vi "Nicolet 12 ICAI_gatefix4.vi"(3 "?":u16(ring)=10 items=["16", "32", "64", "128", "256", "512", "1024", "2048", "4096", "8192", "16384", "32768", "65536", "131072", "262144", "524288 (one channel)", ""], 5 "Sample Duration (sec)":u32(knob)=24 scale=1.0..33.0) -> (0 "Waveform Graph":waveform(dbl)[](graph)=[{"t0"=timestamp(0 s since 1904-01-01), "dt"=0.0001220703125, "Y"=array[40960 elements]}, {"t0"=timestamp(0 s since 1904-01-01), "dt"=0.0001220703125, "Y"=array[40960 elements]}], 2 "data":dbl[][](array[numeric]) format="%0.2f", 8 "points":i32=40960)   [LabVIEW 2010]
doc: "I. Description:\nThis example demonstrates how to acquire a finite amount of data (Waveform) using the DAQ device's internal clock, started by an analog edge condition.\n\nII. Instructions for Running:\n1. Select the physical channel to correspond to where your signal is input on the DAQ device.\n2. Enter the minimum and maximum voltage range.\nNote: For better accuracy try to match the input range to the expected voltage level of the measured signal.\n3. Set the number of samples to acquire per channel.\n4. Set the rate of the acquisition\nNote: The rate should be AT LEAST twice as fast as the maximum frequency component of the signal being acquired.\n5. Set the source of the start trigger. By default this is PFI0\n6. Set the slope and level of desired analog edge condition.\n\nIII. Block Diagram Steps:\n1. Create an empty task.\n2. Create an analog input voltage channel.\n3. Set the rate for the sample clock. Additionally, define the sample mode to be finite.\n4. Define the parameters for an Analog Slope Start Trigger.\n5. Call the Start VI to start the acquisition.\n6. Read all of the data.\n7. Stop the Analog Input Task.\n8. Call the Clear Task VI to clear the Task.\n9. Use the popup dialog box to display an error if any\nIV. I/O Connections Overview:\nMake sure your signal input terminal matches the Physical Channel I/O Control. In this case wire your signal to the ai0 pin on your DAQ Device."
uses:
  programs/Detection/200262.llb/Trigger Select.ctl
  <vilib>/Utility/error.llb/DialogType.ctl
  <vilib>/DAQmx/read.llb/DAQmx Read (Analog 2D DBL NChan NSamp).vi
  <vilib>/DAQmx/create/channels.llb/DAQmx Create Channel (AI-Voltage-Basic).vi
  <vilib>/DAQmx/configure/timing.llb/DAQmx Timing (Sample Clock).vi
  <vilib>/DAQmx/configure/trigger.llb/DAQmx Start Trigger (Analog Edge).vi
  <vilib>/DAQmx/configure/trigger.llb/DAQmx Reference Trigger (Digital Edge).vi
  <vilib>/daqmx/miscellaneous.llb/DAQmx Fill In Error Info.vi
  Program Files/National Instruments/LabVIEW 2010/resource/objmgr/daqmx.rc
  <instrlib>/BK Precision 911X Series/BK Precision 911X Series.lvlib
panel:
  in  "Final Current":dbl=16.5
  in  "Current Step (0.0A":dbl=0.02
  in  "Starting Current (0.0 A)":dbl=18.0 format="%.3g"
  in  "Voltage Level (0.0 V)":dbl=15.0 format="%.3f"
  in  "Enable OVP (T: Enable)":bool=TRUE
  in  "Voltage Limit (0V)":dbl=25.0 format="%.2f"
  in  "Magnet Supply VISA name":refnum<visa-resource-name>="GPIB0::1::INSTR"
  out "size(s)":i32[](array[numeric])
  in  "CAI/ICAI":bool=TRUE
  in  "?":path=path "C:/Users/Cardenas/Desktop/7_01/7_01_380fringe371mvmid_lockedat330.txt"
  in  "Path":path=path "C:/Users/Cardenas/Desktop/Feb_2026/02_13_17Mhz_18a_start_p005fall_500uVsense_10avgs_1750hzcenter_negslope.txt"
  out "Time":dbl=5.5
  out "points pretriger":dbl=4096.0
  in  "Iterations to Average":i32=10
  in  "Sample Rate Hz":bool
  out "Cursor Time Selected":dbl=0.22413589186805782
  out "Cursor Peak to Peak Voltage":dbl=0.01024955436720143
  in  "Save Average To File":bool
  out "Pretrigger Samples":dbl=4096.0
  out "Seconds Per Division":dbl=0.1
  out "Posttrigger Samples Captured":dbl=40960.0
  in  "Voltage Offset":dbl(knob) scale=-2.0..2.0
  in  "Average / Live Display":bool
  in  "Seconds  Per Division":u32(knob) min=1 max=1 step=1 scale=0.0..15.0
  out "Samples Averaged":i32=3
  in  "?":bool=TRUE
  in  "Volts Per Division":dbl(knob)=0.5 scale=0.005..5.0
  in  "Pretrigger Duration (%)":dbl(knob)=0.1 min=0.0 max=2.0 step=1.0 scale=0.05..0.95
  in  "Analog Source":string="APFI0"
  in  "Digital External TTL Source":tag="/Dev1/PFI13"
  in  "Trigger Type":T1=enum."Digital Edge"
  in  "Analog Edge Level":dbl=-0.1 format="%0.2f"
  in  "Edge":i32(ring)=10280 items=["Rising"=10280, "Falling"=10171]
  in  "Physical Channel":tag="Dev1/ai22, Dev1/ai23" caption="Physical Channels"
  out "Sampling Iterations":i32=2
  in  "Maximum  Voltage":dbl=10.0
  in  "Minimum Voltage":dbl=-10.0
  out "Sampling Rate":i32=8192 caption="Sample Rate (Hz)"
  in  "stop":bool
  # "Channel\nConfiguration"
  # "Triggering Parameters"
  # "Voltage Parameters"
  # "TTL Trigger Options"
  # "Timing Parameters"
  # "External  Trigger Options"
  # "Storage Options"
  # "Nicolet 8.vi*If X scale markers are not drawn:\nRight click the waveform diagram -> select X axis -> marker spacing -> set to arbitrary AFTER\nsetting the correct seconds per division"
  # "CAI / ICAI"
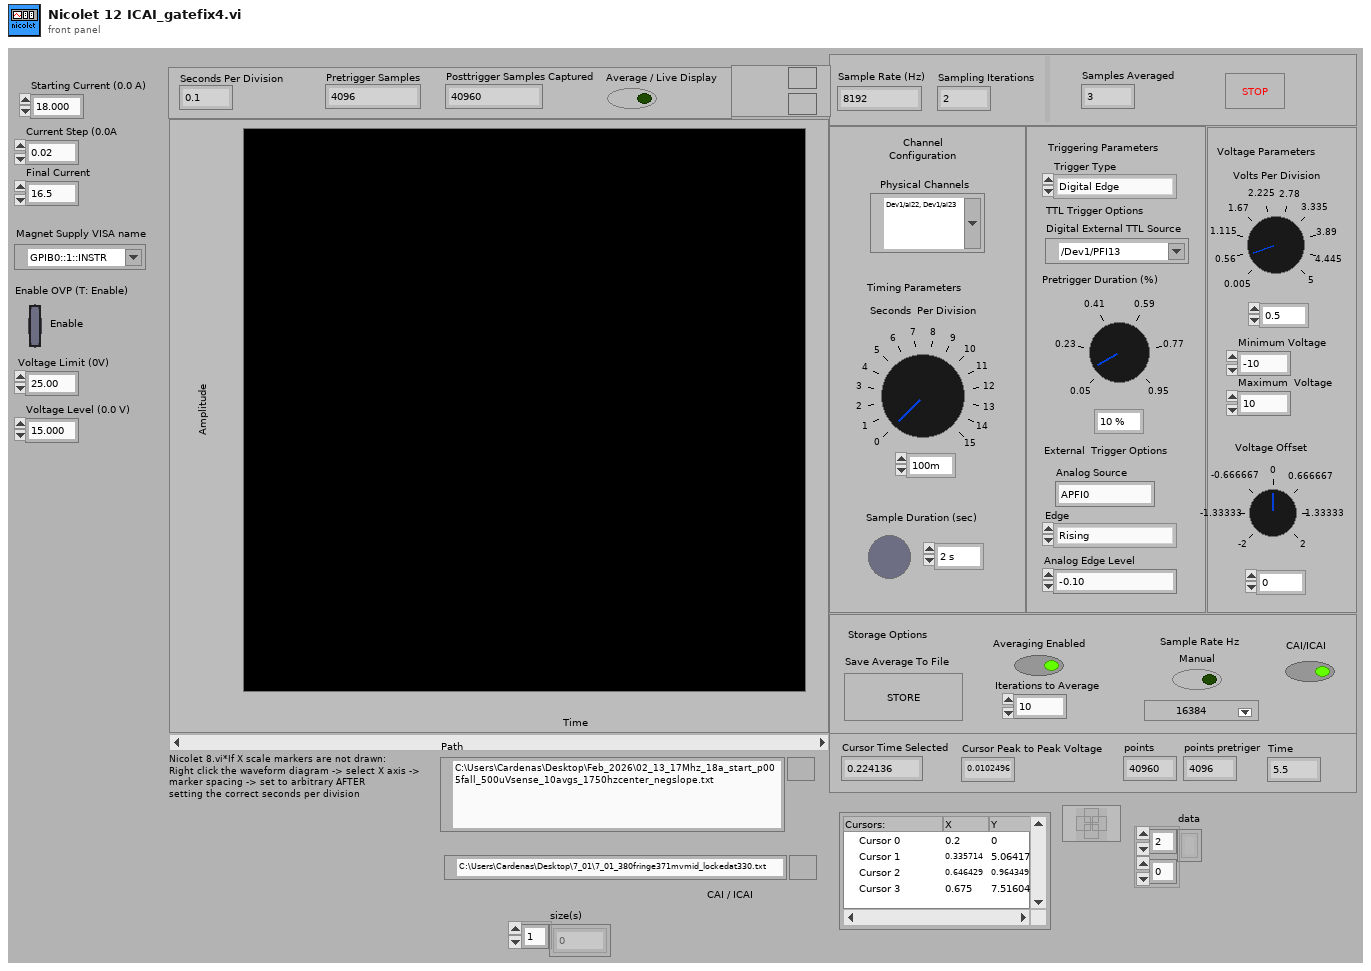
[diagram p1: front panel]
types:
  T1 = typedef "Trigger Select.ctl" = enum16{"None", "Analog Edge", "Digital Edge"}
  T2 = typedef "DialogType.ctl" = u16
  T3 = typedef "LVCursorListTypeDef.ctl" = cluster{"Name":string, "Color":u32, "Style":u8, "Point Style":u8, "Name Visible":bool, "Allow Drag":bool, "Cursor Mode":u32, "Plot":i32, "Index":i32, "Position":cluster{"X":dbl, "Y":dbl}, "X Scale":u32, "Y Scale":u32, "Watch Plots":i32[], "Watch All Plots":bool, "Plot Area":i32, "Label Offset":cluster{"X":dbl, "Y":dbl}}[]
  T4 = cluster{"Name":string, "Color":u32, "Style":u8, "Point Style":u8, "Name Visible":bool, "Allow Drag":bool, "Cursor Mode":u32, "Plot":i32, "Index":i32, "Position":cluster{"X":dbl, "Y":dbl}, "X Scale":u32, "Y Scale":u32, "Watch Plots":i32[], "Watch All Plots":bool, "Plot Area":i32, "Label Offset":cluster{"X":dbl, "Y":dbl}}
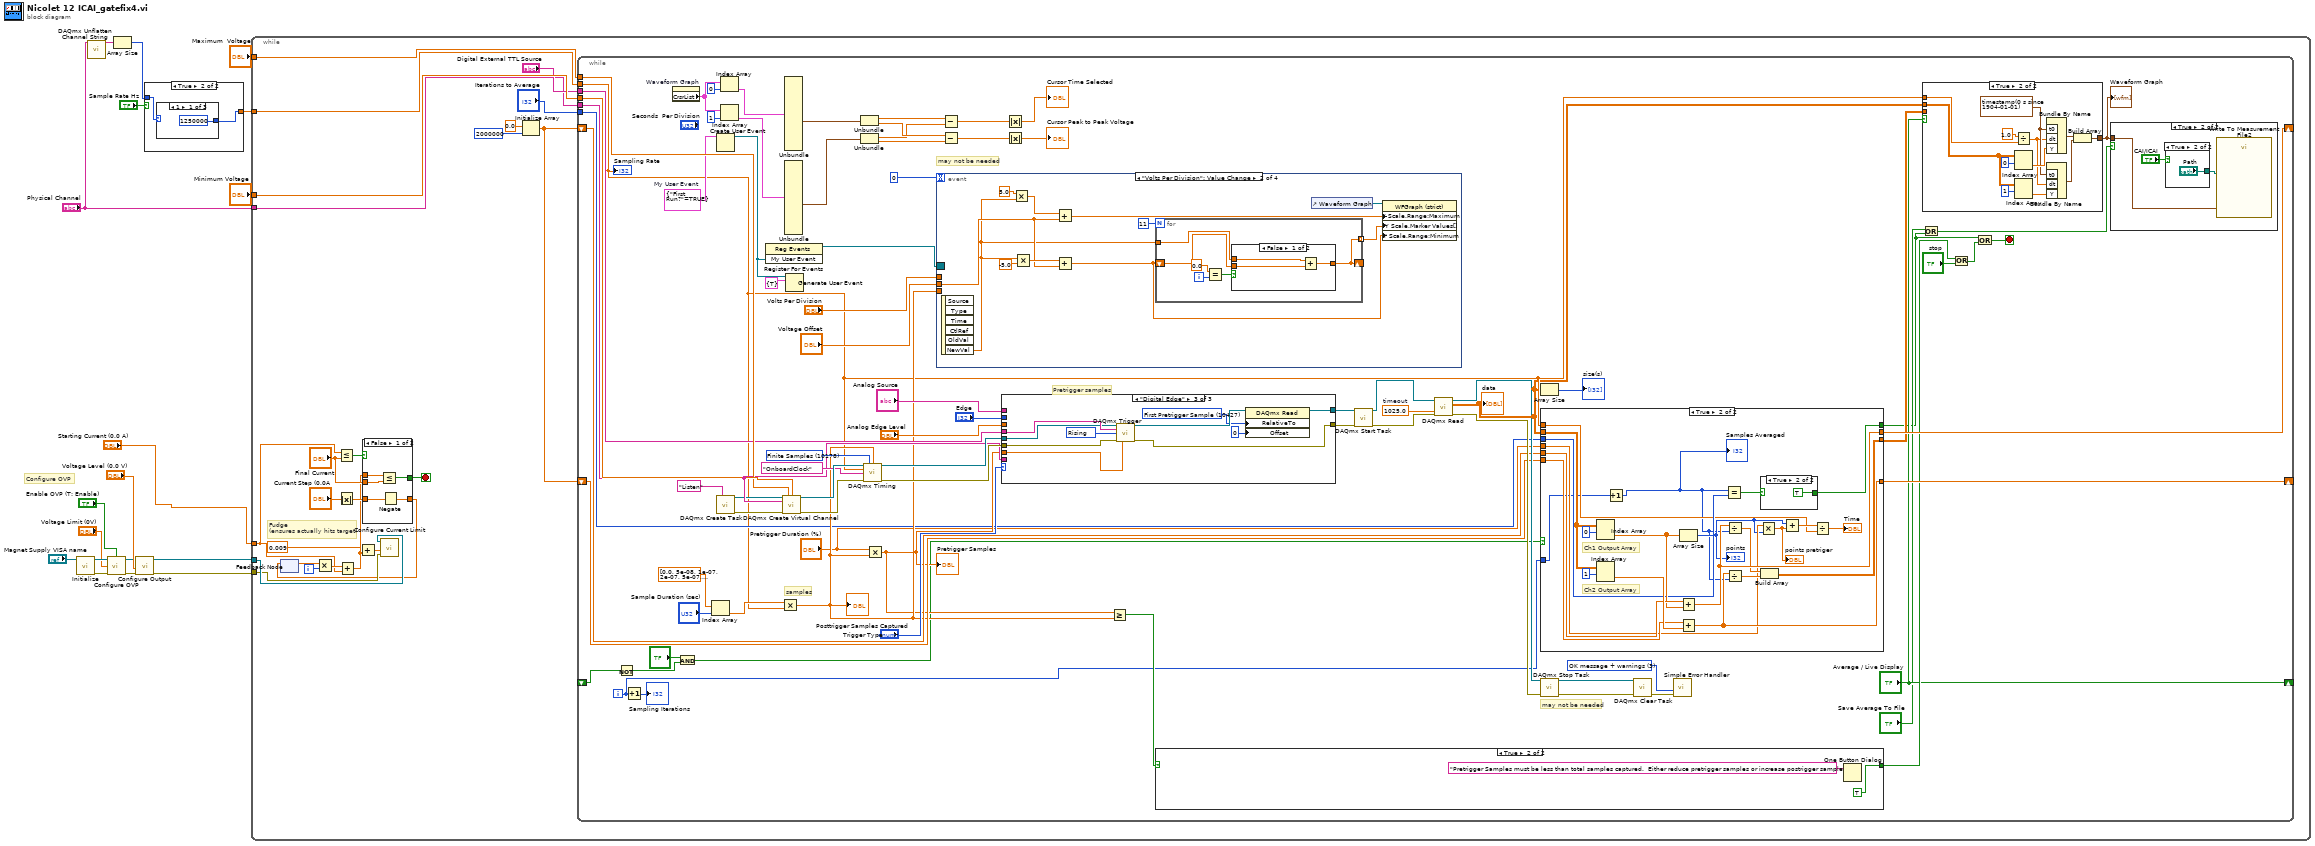
[diagram p0: block diagram]
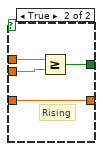
[diagram p2: hidden frame]
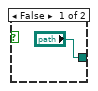
[diagram p4: hidden frame]
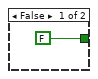
[diagram p5: hidden frame]
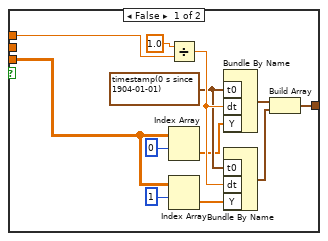
[diagram p6: hidden frame]
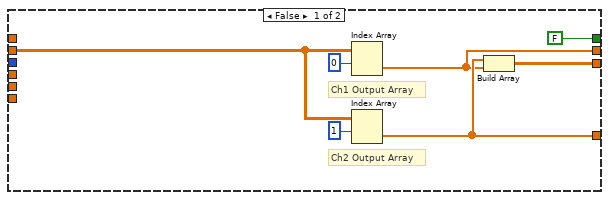
[diagram p7: hidden frame]
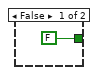
[diagram p8: hidden frame]
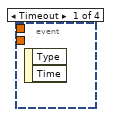
[diagram p9: hidden frame]
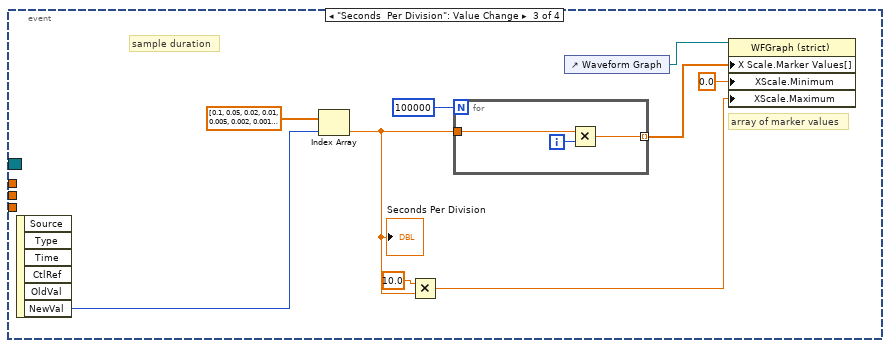
[diagram p11: hidden frame]
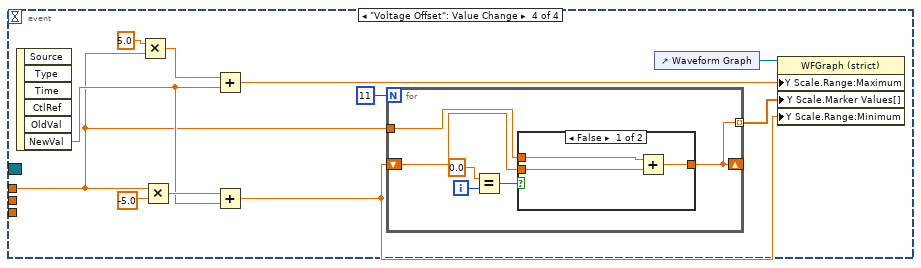
[diagram p12: hidden frame]
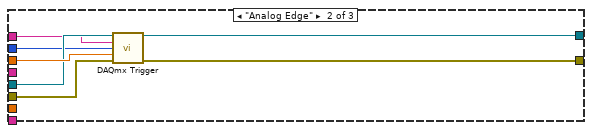
[diagram p15: hidden frame]
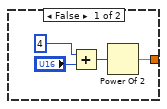
[diagram p16: hidden frame]
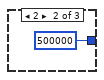
[diagram p17: hidden frame]
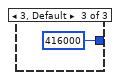
[diagram p18: hidden frame]
diagram:
  # "Configure OVP"
  n1 = call <instrlib>:"Initialize.vi"("VISA resource name"="Magnet Supply VISA name") -> ("error out"=w10:errorcluster, "VISA resource name out"=w9:refnum<visa-resource-name>)  [unwired: 9 in]
  n2 = call <vilib>:"DAQmx Unflatten Channel String.vi"("names in"="Physical Channel") -> ("names out"=w15:string[])  [unwired: 1 in, 13 out]
  n3 = call <instrlib>:"Configure OVP.vi"("VISA resource name"=w9, "Enable OVP (T: Enable)"="Enable OVP (T: Enable)", "Voltage Limit (80.000 V)"="Voltage Limit (0V)", "error in (no error)"=w10) -> ("VISA resource name out"=w5:refnum<visa-resource-name>, "error out"=w4:errorcluster)  [unwired: 10 in]
  n4 = Array Size(array=w15) -> (size(s)=w13:i32)
  n5 = call <instrlib>:"Configure Output.vi"("error in (no error)"=w4, "Voltage Level (0.0 V)"="Voltage Level (0.0 V)", "VISA resource name"=w5) -> ("error out"=w2:errorcluster, "VISA resource name out"=w3:refnum<visa-resource-name>)  [unwired: 7 in]
  n6 = case shown="True" "Sample Rate Hz" {
    tunnel: [w20 w24] -> w14
    tunnel: w13 -> [_ w23]
    frame False {
      n7 = Add(x=4, y="?") -> (x+y=w21:i32)
      n8 = Power Of 2(x=w21) -> (2^x=w20:dbl)
    }
    frame True {
      n9 = case shown="1" w23 {
        tunnel: [1250000 500000 416000] -> w24
        frame 1 {
        }
        frame 2 {
        }
        frame 3, Default {
        }
      }
    }
  }
  n10 = while {
    tunnel: "Minimum Voltage" -> [w51]
    tunnel: "Maximum  Voltage" -> [w50]
    tunnel: "Physical Channel" -> [w48]
    tunnel: w14 -> [w47]
    tunnel: w3 -> [w42]
    tunnel: w2 -> [w41]
    tunnel: "Starting Current (0.0 A)" -> [w36]
    i -> [w33]
    stop <- w39 stop-if-true
    # "Fudge\n(ensures actually hits target)"
    n11 = feedback #1() -> (w34:dbl)  [unwired: 1 in]
    n12 = Multiply(x=w34, y=w33) -> (x*y=w40:dbl)
    n13 = Less Or Equal?(x=w36, y="Final Current") -> (x <= y?=w38:bool)
    n14 = Absolute Value(x="Current Step (0.0A") -> (abs(x)=w31:dbl)
    n15 = Add(x=w40, y=w36) -> (x+y=w30:dbl)
    n16 = Add(x=0.009 ("y"), y=w30) -> (x+y=w28:dbl)
    n17 = case shown="False" w38 {
      tunnel: [w56 w60] -> w39
      tunnel: w30 -> [w55 w59]
      tunnel: "Final Current" -> [w54 w58]
      tunnel: [w52 w57] -> w35
      tunnel: w31 -> [w53 w57]
      frame False {
        n18 = Less Or Equal?(x=w55, y=w54) -> (x <= y?=w56:bool)
        n19 = Negate(x=w53) -> (-x=w52:dbl)
      }
      frame True {
        # "Rising"
        n20 = Greater Or Equal?(x=w59, y=w58) -> (x >= y?=w60:bool)
      }
    }
    n21 = feedback-in #1(w35) -> ()
    n22 = call <instrlib>:"Configure Current Limit.vi"("error in (no error)"=w41, "Current Limit (0.0 A)"=w28, "VISA resource name"=w42) -> ()  [unwired: 7 in, 2 out]
    n23 = Initialize Array(0.0, 2000000) -> (w43:dbl[])
    n24 = while {
      tunnel: w51 -> [w122]
      tunnel: w50 -> [w121]
      tunnel: w48 -> [w120]
      tunnel: "Digital External TTL Source" -> [w118]
      shift-right: [w112] -> _
      shift-left: w43 -> [w111]
      shift-right: [w107] -> _
      shift-left: w43 -> [w106]
      tunnel: w47 -> [w69]
      shift-right: ["Average / Live Display"] -> _
      shift-left: _ -> [w79]
      tunnel: "Iterations to Average" -> [w71]
      i -> [w61]
      stop <- w68 stop-if-true
      w117 = cluster{"First Run?":bool} {"First Run?"=TRUE}  # My User Event
      w137 = T2 3 items=["no dialog", "OK message", "continue or stop message", "OK message + warnings", "continue/stop + warnings"] ("type of dialog (OK msg:1)")
      w134 = 1025.0  # timeout
      w132 = 10178 items=["Finite Samples"=10178, "Continuous Samples"=10123] ("sample mode")
      # "samples"
      # "may not be needed"
      # "may not be needed"
      # "Pretrigger samples"
      n25 = Not(x=w79) -> (.not. x?=w78:bool)
      n26 = Increment(x=w61) -> (x+1=→"Sampling Iterations":i32)
      n27 = property on="Waveform Graph" class="WFGraph (strict)"() -> ("CrsrList"=w75:T3)  [unwired: 2 in, 2 out]
      n28 = And(x="?", y=w78) -> (x .and. y?=w77:bool)
      n29 = Index Array(array=dbl[] [0.0, 5e-08, 1e-07, 2e-07, 5e-07, 1e-06, 2e-06, 5e-06, 1e-05, 2e-05, 5e-05, 0.0001, 0.0002, 0.0005, 0.001, 0.002, 0.005, 0.01, 0.02, 0.05, 0.1, 0.2, 0.5, 1.0, 2.0, 5.0, 10.0, 16.5, 32.5, 65.0, 129.0, 257.0, 513.0, 1025.0], index="Sample Duration (sec)") -> (element=w76:dbl)
      n30 = call <vilib>:"DAQmx Create Task.vi"("new task name"="Listen") -> ("task out"=w110:refnum<k21>, "error out"=w109:errorcluster)  [unwired: 4 in, 9 out]
      n31 = Create User Event(user event datatype=w117) -> (user event=w115:refnum<user-event>)  [unwired: 1 in, 1 out]
      n32 = Index Array(array=w75, index=0) -> (element=w93:T4)
      n33 = Index Array(array=w75, index=1) -> (element=w92:T4)
      n34 = register-events(w115) -> (reference out=w113:refnum<event-registration>)  [unwired: 2 in, 1 out]
      n35 = Multiply(x=w76, y=w69) -> (x*y=w98:dbl)
      "Posttrigger Samples Captured" <- w98
      n36 = call-poly <vilib>:"DAQmx Create Virtual Channel.vi"("task in"=w110, "maximum value"=w121, "minimum value"=w122, "physical channels"=w120, "error in"=w109) -> ("task out"=w133:refnum<k21>, "error out"=w141:errorcluster)  [unwired: 4 in, 5 out]
      n37 = Unbundle(w93) -> ("Position"=w91:cluster{"X":dbl, "Y":dbl})  [unwired: 15 out]
      n38 = Unbundle(w92) -> ("Position"=w90:cluster{"X":dbl, "Y":dbl})  [unwired: 15 out]
      n39 = Generate User Event(user event=w115, event data cluster=cluster{"First Run?":bool} {"First Run?"=TRUE} ("event data")) -> ()  [unwired: 1 in, 2 out]
      n40 = Unbundle(w91) -> ("X"=w85:dbl, "Y"=w89:dbl)
      n41 = Unbundle(w90) -> ("X"=w83:dbl, "Y"=w88:dbl)
      n42 = call-poly <vilib>:"DAQmx Timing.vi"("task/channels in"=w133, "sample mode"=w132, "samples per channel"=w98, "rate"=w69, "source"=tag "OnboardClock", "error in"=w141) -> ("task out"=w127:refnum<k21>, "error out"=w125:errorcluster)  [unwired: 1 in, 7 out]
      n43 = Multiply(x="Pretrigger Duration (%)", y=w98) -> (x*y=w97:dbl)
      "Pretrigger Samples" <- w97
      n44 = event shown="[1] \"Volts Per Division\": Value Change" {
        selector: w113 -> [_ _ _ _]
        dyn-events: _ -> [_ _ _ _]
        timeout: 0 -> [_ _ _ _]
        tunnel: w98 -> [_ _ _ _]
        tunnel: "Voltage Offset" -> [_ w208 _ _]
        tunnel: "Volts Per Division" -> [_ _ _ w240]
        event Timeout {
          n45 = event-data() -> ()  [unwired: 3 out]
        }
        event "Volts Per Division": Value Change {
          n46 = event-data() -> ("NewVal"=w207:dbl)  [unwired: 6 out]
          n47 = Multiply(x=5.0, y=w207) -> (x*y=w212:dbl)
          n48 = Multiply(x=w207, y=-5.0) -> (x*y=w213:dbl)
          n49 = Add(x=w212, y=w208) -> (x+y=w210:dbl)
          n50 = Add(x=w213, y=w208) -> (x+y=w211:dbl)
          n51 = for {
            N: 11 -> [_]
            tunnel: w207 -> [w222]
            tunnel: [w221] -> w209 mode=indexing
            shift-right: [w221] -> _
            shift-left: w211 -> [w219]
            i -> [w217]
            n52 = Equal?(x=0.0, y=w217) -> (x = y?=w220:bool)
            n53 = case shown="False" w220 {
              tunnel: w222 -> [w225 _]
              tunnel: w219 -> [w224 w226]
              tunnel: [w223 w226] -> w221
              frame False {
                n54 = Add(x=w225, y=w224) -> (x+y=w223:dbl)
              }
              frame True {
              }
            }
          }
          n55 = control-ref of="Waveform Graph"() -> (w206:refnum<vi>)
          n56 = property on="Property Node" class="WFGraph (strict)"(reference=w206, "Y Scale.Range:Maximum"=w210, "Y Scale.Marker Values[]"=w209, "Y Scale.Range:Minimum"=w211) -> ()  [unwired: 1 in, 2 out]
        }
        event "Seconds  Per Division": Value Change {
          # "sample duration"
          # "array of marker values"
          n57 = event-data() -> ("NewVal"=w234:u32)  [unwired: 6 out]
          n58 = Index Array(array=dbl[] [0.1, 0.05, 0.02, 0.01, 0.005, 0.002, 0.001, 0.0005, 0.0002, 0.0001, 5e-05, 2e-05, 1e-05, 5e-06, 2e-06, 1e-06], index=w234) -> (element=w228:dbl)
          "Seconds Per Division" <- w228
          n59 = Multiply(x=10.0, y=w228) -> (x*y=w227:dbl)
          n60 = for {
            N: 100000 -> [_]
            tunnel: w228 -> [w237]
            tunnel: [w236] -> w230 mode=indexing
            i -> [w238]
            n61 = Multiply(x=w237, y=w238) -> (x*y=w236:dbl)
          }
          n62 = control-ref of="Waveform Graph"() -> (w232:refnum<vi>)
          n63 = property on="Property Node" class="WFGraph (strict)"(reference=w232, "X Scale.Marker Values[]"=w230, "XScale.Minimum"=0.0 ("x"), "XScale.Maximum"=w227) -> ()  [unwired: 1 in, 2 out]
        }
        event "Voltage Offset": Value Change {
          n64 = event-data() -> ("NewVal"=w241:dbl)  [unwired: 6 out]
          n65 = Multiply(x=5.0, y=w240) -> (x*y=w249:dbl)
          n66 = Multiply(x=w240, y=-5.0) -> (x*y=w248:dbl)
          n67 = Add(x=w249, y=w241) -> (x+y=w244:dbl)
          n68 = Add(x=w248, y=w241) -> (x+y=w242:dbl)
          n69 = for {
            N: 11 -> [_]
            tunnel: w240 -> [w255]
            tunnel: [w254] -> w243 mode=indexing
            shift-right: [w254] -> _
            shift-left: w242 -> [w252]
            i -> [w250]
            n70 = Equal?(x=0.0, y=w250) -> (x = y?=w253:bool)
            n71 = case shown="False" w253 {
              tunnel: w255 -> [w258 _]
              tunnel: w252 -> [w257 w259]
              tunnel: [w256 w259] -> w254
              frame False {
                n72 = Add(x=w258, y=w257) -> (x+y=w256:dbl)
              }
              frame True {
              }
            }
          }
          n73 = control-ref of="Waveform Graph"() -> (w239:refnum<vi>)
          n74 = property on="Property Node" class="WFGraph (strict)"(reference=w239, "Y Scale.Range:Maximum"=w244, "Y Scale.Marker Values[]"=w243, "Y Scale.Range:Minimum"=w242) -> ()  [unwired: 1 in, 2 out]
        }
      }
      n75 = Subtract(x=w85, y=w83) -> (x-y=w84:dbl)
      n76 = Subtract(x=w89, y=w88) -> (x-y=w87:dbl)
      n77 = case shown="\"Digital Edge\"" "Trigger Type" {
        tunnel: w127 -> [w261 w264 w275]
        tunnel: [w261 w266 w271] -> w126
        tunnel: w125 -> [w260 w268 w273]
        tunnel: [w260 w265 w278] -> w124
        tunnel: w120 -> [_ _ _]
        tunnel: "Analog Edge Level" -> [_ w267 _]
        tunnel: "Analog Source" -> [_ w263 _]
        tunnel: w118 -> [_ _ w277]
        tunnel: w97 -> [_ _ w274]
        tunnel: "Edge" -> [_ w262 _]
        frame "None", Default {
        }
        frame "Analog Edge" {
          n78 = call-poly <vilib>:"DAQmx Trigger.vi"("task/channels in"=w264, "source"=w263, "slope"=w262, "level"=w267, "error in"=w268) -> ("task out"=w266:refnum<k21>, "error out"=w265:errorcluster)  [unwired: 9 out]
        }
        frame "Digital Edge" {
          w269 = 10427 items=["First Sample"=10424, "Current Read Position"=10425, "Reference Trigger"=10426, "First Pretrigger Sample"=10427, "Most Recent Sample"=10428] ("RelativeTo")
          w276 = 10280 items=["Rising"=10280, "Falling"=10171] ("edge")
          n79 = call-poly <vilib>:"DAQmx Trigger.vi"("task/channels in"=w275, "source"=w277, "edge"=w276, "error in"=w273, "pretrigger samples per channel"=w274) -> ("task out"=w272:refnum<k21>, "error out"=w278:errorcluster)  [unwired: 9 out]
          n80 = property class="DAQmx Read"(reference=w272, "RelativeTo"=w269, "Offset"=0) -> (reference out=w271:refnum<k21>)  [unwired: 1 in, 1 out]
        }
      }
      n81 = Absolute Value(x=w84) -> (abs(x)=→"Cursor Time Selected":dbl)
      n82 = Absolute Value(x=w87) -> (abs(x)=→"Cursor Peak to Peak Voltage":dbl)
      n83 = Greater Or Equal?(x=w97, y=w98) -> (x >= y?=w101:bool)
      n84 = case shown="True" w101 {
        tunnel: [FALSE TRUE] -> w99
        frame False {
        }
        frame True {
          n85 = One Button Dialog(message="Pretrigger Samples must be less than total samples captured.  Either reduce pretrigger samples or increase postrigger samples.") -> ()  [unwired: 2 out]
        }
      }
      n86 = call <vilib>:"DAQmx Start Task.vi"("task/channels in"=w126, "error in"=w124) -> ("task out"=w135:refnum<k21>, "error out"=w140:errorcluster)  [unwired: 12 out]
      n87 = call-poly <vilib>:"DAQmx Read.vi"("task/channels in"=w135, "timeout"=w134, "error in"=w140) -> ("task out"=w131:refnum<k21>, "data"=w64:dbl[][], "error out"=w130:errorcluster)  [unwired: 1 in, 9 out]
      "data" <- w64
      n88 = Array Size(array=w64) -> (size(s)=→"size(s)":i32[])
      n89 = case shown="True" w77 {
        tunnel: w64 -> [w178 w203]
        tunnel: [w176 w200] -> w112
        tunnel: w111 -> [_ w198]
        tunnel: [w177 w197] -> w107
        tunnel: w106 -> [_ w196]
        tunnel: [w175 w193] -> w96
        tunnel: [FALSE w191] -> w66
        tunnel: w71 -> [_ w189]
        tunnel: "Pretrigger Duration (%)" -> [_ w188]
        tunnel: w69 -> [_ w184]
        tunnel: w61 -> [_ w181]
        frame False {
          # "Ch2 Output Array"
          # "Ch1 Output Array"
          n90 = Index Array(array=w178, index (row)=0 ("disabled index (col)")) -> (element=w176:dbl[])  [unwired: 1 in]
          n91 = Index Array(array=w178, index (row)=1 ("disabled index (col)")) -> (element=w177:dbl[])  [unwired: 1 in]
          n92 = Build Array(w177, w176) -> (w175:dbl[][])
        }
        frame True {
          # "Ch2 Output Array"
          # "Ch1 Output Array"
          n93 = Index Array(array=w203, index (row)=0 ("disabled index (col)")) -> (element=w192:dbl[])  [unwired: 1 in]
          n94 = Index Array(array=w203, index (row)=1 ("disabled index (col)")) -> (element=w199:dbl[])  [unwired: 1 in]
          n95 = Increment(x=w181) -> (x+1=w182:i32)
          "Samples Averaged" <- w182
          n96 = Array Size(array=w192) -> (size(s)=w187:i32)
          "points" <- w187
          n97 = Add(x=w198, y=w192) -> (x+y=w200:dbl[])
          n98 = Add(x=w196, y=w199) -> (x+y=w197:dbl[])
          n99 = Equal?(x=w182, y=w189) -> (x = y?=w190:bool)
          n100 = Divide(x=w200, y=w182) -> (x/y=w195:dbl[])
          n101 = Divide(x=w197, y=w182) -> (x/y=w194:dbl[])
          n102 = Multiply(x=w188, y=w187) -> (x*y=w186:dbl)
          "points pretriger" <- w186
          n103 = case shown="True" w190 {
            tunnel: [FALSE TRUE] -> w191
            frame False {
            }
            frame True {
            }
          }
          n104 = Build Array(w195, w194) -> (w193:dbl[][])
          n105 = Add(x=w187, y=w186) -> (x+y=w185:dbl)
          n106 = Divide(x=w185, y=w184) -> (x/y=→"Time":dbl)
        }
      }
      n107 = call <vilib>:"DAQmx Stop Task.vi"("task/channels in"=w131, "error in"=w130) -> ("task out"=w136:refnum<k21>, "error out"=w139:errorcluster)  [unwired: 12 out]
      n108 = call <vilib>:"DAQmx Clear Task.vi"("task in"=w136, "error in"=w139) -> ("error out"=w138:errorcluster)  [unwired: 13 out]
      n109 = call <vilib>:"Simple Error Handler.vi"("type of dialog (OK msg:1)"=w137, "error in (no error)"=w138) -> ()  [unwired: 8 out]
      n110 = case shown="True" "Average / Live Display" {
        tunnel: w64 -> [_ w170]
        tunnel: [w152 w162] -> w74
        tunnel: w96 -> [w154 _]
        tunnel: w69 -> [w153 w166]
        frame False {
          w159 = timestamp(0 s since 1904-01-01) ("t0")
          n111 = Divide(x=1.0, y=w153) -> (x/y=w161:dbl)
          n112 = Index Array(array=w154, index (row)=0 ("disabled index (col)")) -> (element=w155:dbl[])  [unwired: 1 in]
          n113 = Index Array(array=w154, index (row)=1 ("disabled index (col)")) -> (element=w158:dbl[])  [unwired: 1 in]
          n114 = Bundle By Name("t0"=w159, "dt"=w161, "Y"=w155) -> (w150:waveform(dbl))  [unwired: 1 out]
          n115 = Bundle By Name("t0"=w159, "dt"=w161, "Y"=w158) -> (w151:waveform(dbl))  [unwired: 1 out]
          n116 = Build Array(w150, w151) -> (w152:waveform(dbl)[])
        }
        frame True {
          w168 = timestamp(0 s since 1904-01-01) ("t0")
          n117 = Divide(x=1.0, y=w166) -> (x/y=w165:dbl)
          n118 = Index Array(array=w170, index (row)=0 ("disabled index (col)")) -> (element=w173:dbl[])  [unwired: 1 in]
          n119 = Index Array(array=w170, index (row)=1 ("disabled index (col)")) -> (element=w169:dbl[])  [unwired: 1 in]
          n120 = Bundle By Name("t0"=w168, "dt"=w165, "Y"=w173) -> (w163:waveform(dbl))  [unwired: 1 out]
          n121 = Bundle By Name("t0"=w168, "dt"=w165, "Y"=w169) -> (w164:waveform(dbl))  [unwired: 1 out]
          n122 = Build Array(w163, w164) -> (w162:waveform(dbl)[])
        }
      }
      "Waveform Graph" <- w74
      n123 = Or(x="Save Average To File", y=w66) -> (x .or. y?=w73:bool)
      n124 = Or(x=w99, y="stop") -> (x .or. y?=w67:bool)
      n125 = Or(x=w66, y=w67) -> (x .or. y?=w68:bool)
      n126 = case shown="True" w73 {
        tunnel: w74 -> [_ w144]
        frame False {
        }
        frame True {
          n127 = case shown="True" "CAI/ICAI" {
            tunnel: ["?" "Path"] -> w143
            frame False {
            }
            frame True {
            }
          }
          n128 = call "Write To Measurement File2"("Signals"=w144, "Filename"=w143) -> ()  [unwired: 15 in, 3 out]
        }
      }
      "Sampling Rate" <- w69
    }
  }
